vi "VI Linearisierung v2.vi"() -> ()   [LabVIEW 2020, in "Linearisierung v2.lvlib"] (continued)
      n15 = control-ref of="PrüfgasName 2"() -> (w61:refnum<vi>)
      n16 = control-ref of="PrüfgasName 3"() -> (w62:refnum<vi>)
      n17 = control-ref of="PrüfgasName 4"() -> (w63:refnum<vi>)
      n18 = control-ref of="PrüfgasName 5"() -> (w64:refnum<vi>)
      n19 = control-ref of="PrüfgasName 6"() -> (w65:refnum<vi>)
      n20 = control-ref of="PrüfgasName 7"() -> (w66:refnum<vi>)
      n21 = control-ref of="PrüfgasName 8"() -> (w67:refnum<vi>)
      n22 = control-ref of="PrüfgasName 9"() -> (w68:refnum<vi>)
      n23 = control-ref of="PrüfgasName 10"() -> (w69:refnum<vi>)
      n24 = Build Array ("Array erstellen")(w60, w61, w62, w63, w64, w65, w66, w67, w68, w69) -> (w50:refnum<vi>[])
      n25 = Build Array ("Array erstellen")(w74, w59, w58, w57, w56, w55, w54, w53, w52, w51) -> (w73:refnum<vi>[])
      n26 = control-ref of="Parameterkontrolle:"() -> (w97:refnum<vi>)
      n27 = control-ref of="Parameterkontrolle: 2"() -> (w98:refnum<vi>)
      n28 = control-ref of="Parameterkontrolle: 3"() -> (w99:refnum<vi>)
      n29 = control-ref of="Parameterkontrolle: 4"() -> (w100:refnum<vi>)
      n30 = control-ref of="Parameterkontrolle: 5"() -> (w101:refnum<vi>)
      n31 = control-ref of="Parameterkontrolle: 6"() -> (w102:refnum<vi>)
      n32 = control-ref of="Parameterkontrolle: 7"() -> (w103:refnum<vi>)
      n33 = control-ref of="Parameterkontrolle: 8"() -> (w104:refnum<vi>)
      n34 = control-ref of="Parameterkontrolle: 9"() -> (w105:refnum<vi>)
      n35 = control-ref of="Parameterkontrolle: 10"() -> (w106:refnum<vi>)
      n36 = control-ref of="Abfragen"() -> (w95:refnum<vi>)
      n37 = control-ref of="Abfragen 2"() -> (w94:refnum<vi>)
      n38 = control-ref of="Abfragen 3"() -> (w93:refnum<vi>)
      n39 = control-ref of="Abfragen 4"() -> (w92:refnum<vi>)
      n40 = control-ref of="Abfragen 5"() -> (w91:refnum<vi>)
      n41 = control-ref of="Abfragen 6"() -> (w90:refnum<vi>)
      n42 = control-ref of="Abfragen 7"() -> (w89:refnum<vi>)
      n43 = control-ref of="Abfragen 8"() -> (w88:refnum<vi>)
      n44 = control-ref of="Abfragen 9"() -> (w87:refnum<vi>)
      n45 = control-ref of="Abfragen 10"() -> (w86:refnum<vi>)
      n46 = control-ref of="auto Scan Points"() -> (w84:refnum<vi>)
      n47 = control-ref of="auto Scan Points 2"() -> (w83:refnum<vi>)
      n48 = control-ref of="auto Scan Points 3"() -> (w82:refnum<vi>)
      n49 = control-ref of="auto Scan Points 4"() -> (w81:refnum<vi>)
      n50 = control-ref of="auto Scan Points 5"() -> (w80:refnum<vi>)
      n51 = control-ref of="auto Scan Points 6"() -> (w79:refnum<vi>)
      n52 = control-ref of="auto Scan Points 7"() -> (w78:refnum<vi>)
      n53 = control-ref of="auto Scan Points 8"() -> (w77:refnum<vi>)
      n54 = control-ref of="auto Scan Points 9"() -> (w76:refnum<vi>)
      n55 = control-ref of="auto Scan Points 10"() -> (w75:refnum<vi>)
      n56 = control-ref of="Stufen Tabelle"() -> (w108:refnum<vi>)
      n57 = control-ref of="Stufen Tabelle 2"() -> (w109:refnum<vi>)
      n58 = control-ref of="Stufen Tabelle 3"() -> (w110:refnum<vi>)
      n59 = control-ref of="Stufen Tabelle 4"() -> (w111:refnum<vi>)
      n60 = control-ref of="Stufen Tabelle 5"() -> (w112:refnum<vi>)
      n61 = control-ref of="Stufen Tabelle 6"() -> (w113:refnum<vi>)
      n62 = control-ref of="Stufen Tabelle 7"() -> (w114:refnum<vi>)
      n63 = control-ref of="Stufen Tabelle 8"() -> (w115:refnum<vi>)
      n64 = control-ref of="Stufen Tabelle 9"() -> (w116:refnum<vi>)
      n65 = control-ref of="Stufen Tabelle 10"() -> (w117:refnum<vi>)
      n66 = Build Array ("Array erstellen")(w84, w83, w82, w81, w80, w79, w78, w77, w76, w75) -> (w72:refnum<vi>[])
      n67 = Build Array ("Array erstellen")(w95, w94, w93, w92, w91, w90, w89, w88, w87, w86) -> (w85:refnum<vi>[])
      n68 = Build Array ("Array erstellen")(w108, w109, w110, w111, w112, w113, w114, w115, w116, w117) -> (w107:refnum<vi>[])
      n69 = Build Array ("Array erstellen")(w97, w98, w99, w100, w101, w102, w103, w104, w105, w106) -> (w96:refnum<vi>[])
      n70 = for {
        tunnel: w72 -> [w118] mode=indexing
        n71 = property class="Bool. (strikt)"(reference=w118, "Value"=TRUE ("Wert")) -> (error out=w119:errorcluster)  [unwired: 1 in, 1 out]
        n72 = call <vilib>:"Clear Errors.vi"("error in (no error)"=w119) -> ()  [unwired: 5 in, 2 out]
      }
      n73 = control-ref of="Autolin Hovacal"() -> (w49:refnum<vi>)
      n74 = control-ref of="Bearbeiter"() -> (w71:refnum<vi>)
      n75 = control-ref of="EPA Auswertung"() -> (w47:refnum<vi>)
      n76 = control-ref of="Daten"() -> (w48:refnum<vi>)
      n77 = control-ref of="LIN Filename override"() -> (w42:refnum<vi>)
      n78 = control-ref of="EPA Filename override"() -> (w41:refnum<vi>)
      n79 = control-ref of="File Name LIN"() -> (w46:refnum<vi>)
      n80 = control-ref of="EPA Filename"() -> (w45:refnum<vi>)
      n81 = control-ref of="Gasnummer Generieren"() -> (w43:refnum<vi>)
      n82 = Bundle("File Name LIN"=w46, "EPA Filename"=w45) -> (w44:T101)  [unwired: 1 in]
      n83 = Bundle("LIN Filename override"=w42, "EPA Filename override"=w41) -> (w40:T102)  [unwired: 1 in]
    }
    frame #1 {
      w185 = u16 0 items=["---", "NO (350,3000) LP 191C", "NO2 (150) LP 191C (1of2)", "NO2 (2000) LP 191C (2of2)", "N2O (300) LP 191C (1of2)", "NH3 (300) LP 191C (1of2)", "NH3 (900,3000) LP 191C (2of2)", "HNCO (400) 191C", "H2O% (30) LP 191C", "Formaldehyde (70,500) LP 191C", "CO2 low% (4) LP 191C (2of2)", "CO2% (20) LP 191C (1of2)", "CO (700) LP 191C (1of3)", "CO% (1) LP 191C (2of3)", "Propylene (1000) LP 191C", "Aromatic HC C7 (500) LP 191C", "Ethylene (1000) LP 191C", "CH4 (250) LP 191C (1of2)", "CH4 (5000) LP 191C (2of2)", "Ethane (1000) LP 191C", "Acetylene (1000) LP 191C", "HNO2 (20) 191C", "MeOH (1000) 191C", "CO% (10) LP 191C (3of3)", "Formic Acid (100) 191C", "SO2 (500) LP 191C", "Acetaldehyde (1000) LP 191C", "COS (100) LP 191C", "1,3 butadiene (100) LP 191C", "Oil as Octane (200) LP 191C", "N2O (1000) LP 191C (2of2)", "Propane (200) LP 191C", "NO2 autorange (2000)", "CO autorange (100000)", "CH4 autorange (5000)", "NH3 autorange (3000)", "NOx autorange (3000)", "HCD (10000)", "NMHCD (10000)", "CO2% autorange (20)", "H2Oppm (300000)", "N2O autorange (1000)", "NMNEHCD (3000)", "Temp. Gascell", "Pressure Gascell", "sBeam@2500", "Temp. HL zu FT-IR", "Temp. HL Extern SP1", "Austrittstemp. FT-IR", "Temp. Schaltschrank", "Konstant 0", "Konstant 50", "Konstant 100", "AK DUMMY"] ("passive Komponente:")
      # "#RickQuickTest_Features"
      # "#STB_keep"
      # "#LIN_only_saved_Polynoms"
      # "#PDF_manu_MG"
      # "Daten aufzeichnen"
      # "LIN"
      # "init Analysatoren"
      # "immer auf dieser Seite bleiben ?!"
      # "#Option10xSpanAuto"
      n84 = control-ref of="Hauptregisterkarte"() -> (w211:refnum<vi>)
      n85 = control-ref of="SpanRegister"() -> (w271:refnum<vi>)
      n86 = call "FGV Spans abarbeiten.vi"("Aktion"=Aktion_FGV_Spans_abarbeiten."init") -> ("error out"=w153:errorcluster)  [unwired: 5 in, 5 out]
      n87 = control-ref of="Polynom"() -> (w142:refnum<vi>)
      n88 = control-ref of="Istwerte Abholen"() -> (w251:refnum<vi>)
      n89 = control-ref of="Istwerte löschen"() -> (w252:refnum<vi>)
      n90 = control-ref of="Alles löschen"() -> (w253:refnum<vi>)
      n91 = control-ref of="STARTEN"() -> (w254:refnum<vi>)
      n92 = control-ref of="Speichern LIN"() -> (w165:refnum<vi>)
      n93 = control-ref of="EPA PDF erzeugen"() -> (w164:refnum<vi>)
      n94 = control-ref of="LIN Filename override"() -> (w122:refnum<vi>)
      n95 = control-ref of="EPA Filename override"() -> (w121:refnum<vi>)
      n96 = control-ref of="Spanfactor"() -> (w151:refnum<vi>)
      n97 = control-ref of="Offset"() -> (w150:refnum<vi>)
      n98 = control-ref of="Span 1"() -> (w265:refnum<vi>)
      n99 = control-ref of="Span 2"() -> (w264:refnum<vi>)
      n100 = control-ref of="Span 3"() -> (w263:refnum<vi>)
      n101 = control-ref of="Span 4"() -> (w262:refnum<vi>)
      n102 = control-ref of="Span 5"() -> (w261:refnum<vi>)
      n103 = control-ref of="Span 6"() -> (w260:refnum<vi>)
      n104 = control-ref of="Span 7"() -> (w259:refnum<vi>)
      n105 = control-ref of="Span 8"() -> (w258:refnum<vi>)
      n106 = control-ref of="Span 9"() -> (w257:refnum<vi>)
      n107 = control-ref of="Span 10"() -> (w256:refnum<vi>)
      n108 = control-ref of="HovaCAL MFC1 Komponente:"() -> (w175:refnum<vi>)
      n109 = control-ref of="HovaCAL MFC2 Komponente:"() -> (w174:refnum<vi>)
      n110 = control-ref of="HovaCAL MFC3 Komponente:"() -> (w173:refnum<vi>)
      n111 = control-ref of="HovaCAL MFC4 Komponente:"() -> (w172:refnum<vi>)
      n112 = control-ref of="HovaCAL MFC5 Komponente:"() -> (w171:refnum<vi>)
      n113 = control-ref of="HovaCAL Pump1 Komponente:"() -> (w170:refnum<vi>)
      n114 = control-ref of="HovaCAL Pump2 Komponente:"() -> (w169:refnum<vi>)
      n115 = Build Array(w265, w264, w263, w262, w261, w260, w259, w258, w257, w256) -> (w296:refnum<vi>[])
      n116 = control-ref of="Gasnummer Generieren"() -> (w250:refnum<vi>)
      n117 = control-ref of="Gasnummer HovaCal Interface"() -> (w248:refnum<vi>)
      n118 = control-ref of="Gasnummer HovaCal"() -> (w249:refnum<vi>)
      n119 = control-ref of="Gasnummer LIN"() -> (w163:refnum<vi>)
      n120 = control-ref of="Gasnummer EPA"() -> (w162:refnum<vi>)
      n121 = Bundle("Spanfactor"=w151, "Offset"=w150, "Polynom"=w142) -> (w146:T103)  [unwired: 1 in]
      n122 = control-ref of="passive Komponente:"() -> (w186:refnum<vi>)
      n123 = Bundle("Hauptregisterkarte"=w211, "SpanRegister"=w271) -> (w212:T104)  [unwired: 1 in]
      n124 = Build Array(w251, w252, w253, w254, w165, w164, w122, w121) -> (w244:refnum<vi>[])
      n125 = call "ClusterReferernzenAufschluesseln.vi"("Cluster in"=w296) -> ("error out"=w287:errorcluster, "Analysatoren"=w166:refnum<vi>[], "Ring Gasflasche aktiv out"=w167:refnum<vi>[], "Ring Components out"=w288:refnum<vi>[])  [unwired: 7 in]
      n126 = call "FGV SpanEinstellungen.vi"("Aktion"=Aktion_FGV_SpanEinstellungen."RegisterRef", "error in (no error)"=w153, "RegisterRefs"=w212) -> ("error out"=w239:errorcluster)  [unwired: 4 in, 4 out]
      n127 = disable-structure shown="Aktiviert" {
        disable-tunnel: w165 -> [w303 _]
        disable-tunnel: w164 -> [w302 _]
        disable-tunnel: w163 -> [w301 w306]
        disable-tunnel: w162 -> [w300 w305]
        disable-tunnel: [w299 w304] -> w161
        disable-tunnel: w122 -> [w298 _]
        disable-tunnel: w121 -> [w297 _]
        frame Enabled {
          # "#LinV2_auto_singleSave"
          n128 = Build Array(w298, w297, w303, w302, w301, w300) -> (w299:refnum<vi>[])
        }
        frame Disabled {
          n129 = Build Array(w306, w305) -> (w304:refnum<vi>[])
        }
      }
      n130 = Build Array(w175, w174, w173, w172, w171, w170, w169) -> (w168:refnum<vi>[])
      n131 = Build Array (concatenate)(w168, w186, w288) -> (w187:refnum<vi>[])
      n132 = local write "passive Komponente:"(w185) -> ()
      n133 = Build Array(w250, w248, w249, w163, w162) -> (w243:refnum<vi>[])
      n134 = call "FGV Gasbottledefinition.vi"("Aktion"=Aktion_FGV_Gasbottledefinition."lesen") -> ("Gasflaschen Liste gesamt"=w286:T105[])  [unwired: 8 in, 2 out]
      n135 = call "FGV SpanEinstellungen.vi"("Aktion"=Aktion_FGV_SpanEinstellungen."laden", "error in (no error)"=w239) -> ("error out"=w266:errorcluster, "Punkte umkehren und PDF Optionen Cluster"=w201:T109)  [unwired: 5 in, 3 out]
      n136 = for {
        tunnel: w286 -> [w327]
        tunnel: w167 -> [w325] mode=indexing
        tunnel: [w325] -> w284 mode=indexing
        n137 = call "Gasflaschen Auswahl.vi"("Gasflaschen Liste gesamt"=w327, "Ring (Eingang)"=w325) -> ("error out"=w326:errorcluster)  [unwired: 7 in, 2 out]
        n138 = call <vilib>:"Clear Errors.vi"("error in (no error)"=w326) -> ()  [unwired: 5 in, 2 out]
      }
      n139 = Unbundle By Name(w201) -> ("Punkte umkehren"=w200:bool[], "PDF Optionen"=w199:T108)
      n140 = call "FGV Gasliste.vi"("Aktionen"=FGV_FT-IR_Gasliste_Aktionen."lesen") -> ("Aktuelle Gasliste gesamt"=w292:T48[])  [unwired: 8 in, 2 out]
      n141 = control-ref of="EPA Optionsfeld"() -> (w144:refnum<vi>)
      n142 = call "FGV Komponentenreferenzen verwalten.vi"("Referenzen"=w187, "error in (no error)"=w287, "Aktion"=Aktion_FGV_Komponentenreferenz_verwalten."Referenzen init") -> ("error out"=w289:errorcluster)  [unwired: 12 in]
      n143 = control-ref of="Polynomkoeffizienten"() -> (w141:refnum<vi>)
      n144 = control-ref of="Komponente Daten Gen"() -> (w245:refnum<vi>)
      n145 = control-ref of="Komponentenanzeige LIN"() -> (w246:refnum<vi>)
      n146 = control-ref of="Komponentenanzeige EPA"() -> (w247:refnum<vi>)
      n147 = control-ref of="Einheit"() -> (w192:refnum<vi>)
      n148 = control-ref of="Einheit Deviation"() -> (w191:refnum<vi>)
      n149 = control-ref of="Polynom-Ordnung"() -> (w149:refnum<vi>)
      n150 = control-ref of="Spanfactor LIN"() -> (w148:refnum<vi>)
      n151 = control-ref of="Offset LIN"() -> (w147:refnum<vi>)
      n152 = call "FGV SpanEinstellungen.vi"("Aktion"=Aktion_FGV_SpanEinstellungen."init", "error in (no error)"=w266) -> ("error out"=w268:errorcluster, "SpanInletClusterArray out"=w269:T19[])  [unwired: 5 in, 3 out]
      n153 = Build Array (concatenate)("---" ("String"), w292) -> (w294:T48[])
      n154 = control-ref of="EPA Optionsfeld"() -> (w160:refnum<vi>)
      n155 = control-ref of="Autolin Hovacal"() -> (w206:refnum<vi>)
      n156 = Build Array(w245, w246, w247) -> (w190:refnum<vi>[])
      n157 = Build Array(w192, w191) -> (w189:refnum<vi>[])
      n158 = call "FGV SpanEinstellungen.vi"("Aktion"=Aktion_FGV_SpanEinstellungen."schreiben", "error in (no error)"=w268, "SpanInletClusterArray in"=w269) -> ("error out"=w222:errorcluster, "SpanInletClusterArray out"=w223:T19[])  [unwired: 4 in, 3 out]
      n159 = control-ref of="Bearbeiter"() -> (w210:refnum<vi>)
      n160 = Bundle("Polynom-Ordnung"=w149, "Spanfactor LIN"=w148, "Offset LIN"=w147, "Polynomkoeffizienten"=w141) -> (w145:T110)  [unwired: 1 in]
      n161 = control-ref of="Modus"() -> (w204:refnum<vi>)
      n162 = call "FGV Komponentenreferenzen verwalten.vi"("Strings []"=w294, "error in (no error)"=w289, "Aktion"=Aktion_FGV_Komponentenreferenz_verwalten."Ring beschreiben") -> ("error out"=w214:errorcluster)  [unwired: 12 in]
      n163 = control-ref of="Kalibrierauswahl"() -> (w209:refnum<vi>)
      n164 = control-ref of="Conditions:"() -> (w208:refnum<vi>)
      n165 = control-ref of="HovaCAL AutoLin MFC"() -> (w207:refnum<vi>)
      n166 = Unbundle By Name(w199) -> ("PDF Einzelseiten Komponenten"=w152:bool, "PDF Einzelseiten Span"=w125:bool, "PDF Deckblatt"=w198:bool, "PDF öffnen"=w197:bool, "Graphik für Messwerte"=w129:bool)
      n167 = for {
        tunnel: w203 -> [w317] mode=indexing
        tunnel: w200 -> [w316] mode=indexing
        tunnel: [w315] -> w202 mode=indexing
        n168 = property class="Bool. (strikt)"(reference=w317, "Value"=w316) -> (reference out=w315:refnum<vi>, error out=w318:errorcluster)  [unwired: 1 in]
        n169 = call <vilib>:"Clear Errors.vi"("error in (no error)"=w318) -> ()  [unwired: 5 in, 2 out]
      }
      n170 = call "get first active SPAN.vi"("error in (no error)"=w222, "SpanInletClusterArray in"=w223) -> ("error out"=w220:errorcluster, "Index first active SPAN"=w219:i32, "SpanInletClusterArray out"=w221:T19[])  [unwired: 7 in]
      n171 = Build Array(w210, w160, w209, w208, w207, w206, w204) -> (w205:refnum<vi>[])
      n172 = Bundle(w190, w189, w146, w145, "EPA Optionsfeld"=w144) -> (w143:T111)  [unwired: 1 in]
      n173 = call "get SPAN first active component.vi"("error in (no error)"=w220, "SPAN Idx"=w219, "SpanInletClusterArray in"=w221) -> ("error out"=w213:errorcluster, "first aktive Komponente"=w216:i32, "SPAN Idx out"=w217:i32, "SpanInletClusterArray out"=w218:T19[])  [unwired: 5 in]
      n174 = control-ref of="post processing done"() -> (w178:refnum<vi>)
      n175 = control-ref of="post processing PDFs"() -> (w134:refnum<vi>)
      n176 = control-ref of="passive Komponente:"() -> (w188:refnum<vi>)
      n177 = control-ref of="post processing"() -> (w183:refnum<vi>)
      n178 = Build Array (concatenate)(w161, w160) -> (w159:refnum<vi>[])
      n179 = control-ref of="Eingabetabelle"() -> (w155:refnum<vi>)
      n180 = control-ref of="post processing done"() -> (w176:refnum<vi>)
      n181 = control-ref of="post processing PDFs"() -> (w133:refnum<vi>)
      n182 = call "Set actual ProtocolData from SPAN.vi"("Punkte umkehren Array"=w202, "error in (no error)"=w213, "Comp Idx"=w216, "Index in"=w217, "SpanInletClusterArray in"=w218) -> ("error out"=w156:errorcluster, "SpanInletClusterArray out"=w158:T19[])  [unwired: 3 in, 2 out]
      n183 = control-ref of="post processing"() -> (w179:refnum<vi>)
      n184 = Bundle("passive Komponente:"=w188, "post processing"=w183, "post processing done"=w178, "post processing PDFs"=w134) -> (w184:T112)  [unwired: 1 in]
      n185 = call "FGV SPAN Verriegelung.vi"("Processing Cluster"=w184, "Lin Param Elements Array"=w205, "aktion"=Aktion_FGV_SPAN_Verriegelung."setrefs", "error in (no error)"=w239, "Components Array"=w243, "Buttons Array"=w244, "Set Component Cluster"=w143) -> ("error out"=w240:errorcluster)  [unwired: 2 in, 2 out]
      n186 = call "Init Tables.vi"("error in (no error)"=w156, "Eingabetabelle"=w155, "Index in"=0, "SpanInletClusterArray in"=w158) -> ("SpanInletCluster out"=w157:T19[])  [unwired: 4 in, 3 out]
      n187 = call "FGV SPAN Verriegelung.vi"("aktion"=Aktion_FGV_SPAN_Verriegelung."unlock", "error in (no error)"=w240) -> ("error out"=w139:errorcluster)  [unwired: 7 in, 2 out]
      n188 = Select(t=w129, s=w125, f=T1 FALSE ("t")) -> (s? t:f=w130:T1)
      n189 = for {
        tunnel: w284 -> [w323] mode=indexing
        tunnel: w157 -> [w322] mode=indexing
        shift-right: [w320] -> w215
        shift-left: w214 -> [w319]
        n190 = Unbundle By Name(w322) -> ("Konfig Gasflasche"=w321:T20)
        n191 = call "Konfig Gasflasche aktiv.vi"("error in (no error)"=w319, "Konfig Gasflasche"=w321, "Referenz Gasflasche"=w323) -> ("error out"=w324:errorcluster)  [unwired: 8 in]
        n192 = call <vilib>:"Clear Errors.vi"("error in (no error)"=w324) -> ("error out"=w320:errorcluster)  [unwired: 5 in, 1 out]
      }
      n193 = call "FGV Gasteilerliste laden.vi"("Aktion"=Aktion_FGV_Gasteilerliste_laden."laden", "error in (no error)"=w215) -> ("error out"=w224:errorcluster)  [unwired: 7 in, 2 out]
      n194 = call "FGV Gasteilerliste laden.vi"("Aktion"=Aktion_FGV_Gasteilerliste_laden."Liste erstellen", "error in (no error)"=w224) -> ("error out"=w237:errorcluster)  [unwired: 7 in, 2 out]
      n195 = call "get Summenformeln and update.vi"("Fehler (Eingang, kein Fehler)"=w237, "SpanInletClusterArray in"=w223) -> ("error out"=w193:errorcluster, "ident"=w196:bool, "Summenformeln 1.Komponente"=w236:T12[], "SpanInletClusterArray out"=w195:T19[])  [unwired: 6 in]
      n196 = case shown="False" w196 {
        tunnel: w195 -> [w311 w314]
        tunnel: [w309 w314] -> w194
        tunnel: w193 -> [w307 _]
        frame False {
          n197 = call "FGV SpanEinstellungen.vi"("Aktion"=Aktion_FGV_SpanEinstellungen."schreiben", "error in (no error)"=w307, "SpanInletClusterArray in"=w311) -> ("error out"=w308:errorcluster, "SpanInletClusterArray out"=w310:T19[])  [unwired: 4 in, 3 out]
          n198 = call "FGV SpanEinstellungen.vi"("Aktion"=Aktion_FGV_SpanEinstellungen."speichern", "error in (no error)"=w308, "SpanInletClusterArray in"=w310) -> ("SpanInletClusterArray out"=w309:T19[])  [unwired: 4 in, 4 out]
        }
        frame True {
        }
      }
      n199 = Bundle("post processing"=w179, "post processing done"=w176, "post processing PDFs"=w133) -> (w177:T113)  [unwired: 1 in]
      n200 = call "FGV Post Processing.vi"("LIN/EPA Refs Array"=w159, "Aktion"=Aktion_FGV_Post_Processing."set ref", "Refs Cluster"=w177) -> ("error out"=w180:errorcluster)  [unwired: 5 in, 3 out]
      n201 = local write "PDF single pages Components"(w152) -> ()
      n202 = local write "PDF single pages Span"(w125) -> ()
      n203 = local write "PDF Deckblatt"(w198) -> ()
      n204 = local write "PDF öffnen"(w197) -> ()
      n205 = local write "Graphik für Messwerte"(w130) -> ()
      n206 = call "LIN Polynom Ordnung je Komponente für Protokoll.vi"("Aktion"=Aktion_LIN_Polynom_Ordnung_je_Komponente_für_Protokoll."init initial", "error in (no error)"=w139, "Index in"=T69 {"active SPAN Idx"=0, "active Component Index"=0}) -> ("error out"=w136:errorcluster)  [unwired: 2 in, 6 out]
      n207 = call "FGV Post Processing.vi"("Aktion"=Aktion_FGV_Post_Processing."reset", "error in (no error)"=w180) -> ()  [unwired: 6 in, 4 out]
      n208 = call "LIN Polynom Ordnung oder Aktiv Changes für Postprocessing.vi"("Aktion"=Aktion_LIN_Polynom_Ordnung_ode_Aktiv_Changes_für_Postprocessing."init initial", "error in (no error)"=w136, "active SPAN Idx"=0) -> ("error out"=w132:errorcluster)  [unwired: 5 in, 3 out]
      n209 = call "FGV SPAN Stufentabellen.vi"("Aktion"=Aktion_FGV_SPAN_Stufentabellen."init", "error in (no error)"=w132) -> ()  [unwired: 5 in, 4 out]
      n210 = Index Array(array=w194) -> (element #1=w281:T19, element #2=w280:T19, element #3=w279:T19, element #4=w278:T19, element #5=w277:T19, element #6=w276:T19, element #7=w275:T19, element #8=w274:T19, element #9=w273:T19, element #10=w272:T19)  [unwired: 10 in]
      n211 = Index Array(array=w236) -> (element #1=w235:T12, element #2=w234:T12, element #3=w233:T12, element #4=w232:T12, element #5=w231:T12, element #6=w230:T12, element #7=w229:T12, element #8=w228:T12, element #9=w227:T12, element #10=w226:T12)  [unwired: 10 in]
      n212 = Select(t=T66."Enabled", s=w125, f=T66."Disabled and Grayed Out" ("Deaktiviert")) -> (s? t:f=w123:T66)
      n213 = property on="Graphik für Messwerte" class="Bool. (strikt)"("DisabledEnum"=w123) -> (error out=w124:errorcluster)  [unwired: 2 in, 1 out]
      n214 = local write "Span 1"(w281) -> ()
      n215 = local write "Span 2"(w280) -> ()
      n216 = local write "Span 3"(w279) -> ()
      n217 = local write "Span 4"(w278) -> ()
      n218 = local write "Span 5"(w277) -> ()
      n219 = local write "Span 6"(w276) -> ()
      n220 = local write "Span 7"(w275) -> ()
      n221 = local write "Span 8"(w274) -> ()
      n222 = local write "Span 9"(w273) -> ()
      n223 = local write "Span 10"(w272) -> ()
      n224 = local write "PrüfgasName"(w235) -> ()
      n225 = local write "PrüfgasName 2"(w234) -> ()
      n226 = local write "PrüfgasName 3"(w233) -> ()
      n227 = local write "PrüfgasName 4"(w232) -> ()
      n228 = local write "PrüfgasName 5"(w231) -> ()
      n229 = local write "PrüfgasName 6"(w230) -> ()
      n230 = local write "PrüfgasName 7"(w229) -> ()
      n231 = local write "PrüfgasName 8"(w228) -> ()
      n232 = local write "PrüfgasName 9"(w227) -> ()
      n233 = local write "PrüfgasName 10"(w226) -> ()
      n234 = call <vilib>:"Clear Errors.vi"("error in (no error)"=w124) -> ()  [unwired: 5 in, 2 out]
    }
    frame #2 {
      w373 = FALSE  # sofort HovaCALInterface-Freigabe
      # "#SystemEinstellungenV2 #HovaCALInterface #HovaCALMultiMFC"
      n235 = control-ref of="MFC Output 0"() -> (w336:refnum<vi>)
      n236 = control-ref of="MFC Output 1"() -> (w335:refnum<vi>)
      n237 = control-ref of="MFC Output 2"() -> (w334:refnum<vi>)
      n238 = control-ref of="MFC Output 3"() -> (w333:refnum<vi>)
      n239 = control-ref of="MFC Output 4"() -> (w332:refnum<vi>)
      n240 = control-ref of="Pump Output 1"() -> (w355:refnum<vi>)
      n241 = control-ref of="Pump Output 2"() -> (w354:refnum<vi>)
      n242 = control-ref of="MFC0"() -> (w363:refnum<vi>)
      n243 = control-ref of="MFC1"() -> (w362:refnum<vi>)
      n244 = control-ref of="MFC2"() -> (w361:refnum<vi>)
      n245 = control-ref of="MFC3"() -> (w349:refnum<vi>)
      n246 = control-ref of="MFC4"() -> (w348:refnum<vi>)
      n247 = control-ref of="Pump 1"() -> (w359:refnum<vi>)
      n248 = control-ref of="Pump 2"() -> (w358:refnum<vi>)
      n249 = Build Array(w359, w358) -> (w356:refnum<vi>[])
      n250 = Build Array(w363, w362, w361, w349, w348) -> (w360:refnum<vi>[])
      n251 = control-ref of="Konfig Gasteiler"() -> (w330:refnum<vi>)
      n252 = Build Array(w336, w335, w334, w333, w332) -> (w331:refnum<vi>[])
      n253 = Build Array(w355, w354) -> (w353:refnum<vi>[])
      n254 = call "FGV_HovaCAL_Interface_Kommandos.vi"("Aktion"=Aktion_FGV_HovaCAL_Interface_Kommandos."lesen") -> ("gesammelt ?"=w371:bool)  [unwired: 4 in, 5 out]
      n255 = property on="HovaCALInterface-Freigabe" class="Bool."("Visible"=w371) -> (error out=w370:errorcluster)  [unwired: 2 in, 1 out]
      n256 = call "Gasteiler initialisieren.vi"("Gasteiler Referenz"=w330) -> ()  [unwired: 11 in]
      n257 = call <vilib>:"Clear Errors.vi"("error in (no error)"=w370) -> ()  [unwired: 5 in, 2 out]
      n258 = control-ref of="HovaCAL MFC Gase Cluster 1"() -> (w369:refnum<vi>)
      n259 = control-ref of="HovaCAL MFC Gase Cluster 2"() -> (w368:refnum<vi>)
      n260 = control-ref of="HovaCAL MFC Gase Cluster 3"() -> (w367:refnum<vi>)
      n261 = control-ref of="HovaCAL MFC Gase Cluster 4"() -> (w366:refnum<vi>)
      n262 = control-ref of="HovaCAL MFC Gase Cluster 5"() -> (w365:refnum<vi>)
      n263 = control-ref of="fix+MFC1"() -> (w340:refnum<vi>)
      n264 = control-ref of="fix+MFC2"() -> (w341:refnum<vi>)
      n265 = control-ref of="fix+MFC3"() -> (w342:refnum<vi>)
      n266 = control-ref of="fix+MFC4"() -> (w343:refnum<vi>)
      n267 = control-ref of="fix+MFC5"() -> (w344:refnum<vi>)
      n268 = control-ref of="fix+Pump1"() -> (w345:refnum<vi>)
      n269 = control-ref of="fix+Pump2"() -> (w346:refnum<vi>)
      n270 = control-ref of="Hauptregisterkarte"() -> (w351:refnum<vi>)
      n271 = control-ref of="Cluster.PumpModeGeneral-Cluster"() -> (w381:refnum<vi>)
      n272 = control-ref of="Cluster.Flow Output Cluster (Ausgang)"() -> (w380:refnum<vi>)
      n273 = control-ref of="Cluster.PumpModeGeneral-Cluster 2"() -> (w328:refnum<vi>)
      n274 = control-ref of="HovaCAL Limits Cluster"() -> (w388:refnum<vi>)
      n275 = control-ref of="HovaCAL SetPumpMode"() -> (w387:refnum<vi>)
      n276 = control-ref of="HovaCAL Cluster.PumpModeGeneral"() -> (w386:refnum<vi>)
      n277 = control-ref of="HovaCAL Flow Input Cluster"() -> (w385:refnum<vi>)
      n278 = control-ref of="System Cluster"() -> (w377:refnum<vi>)
      n279 = control-ref of="Cluster.Temp Cluster"() -> (w382:refnum<vi>)
      n280 = control-ref of="Cluster.Pump MassFlow-Cluster"() -> (w379:refnum<vi>)
      n281 = control-ref of="HovaCAL SetPumpMode-Cluster"() -> (w374:refnum<vi>)
      n282 = control-ref of="HovaCAL Temperature"() -> (w384:refnum<vi>)
      n283 = control-ref of="MFC Flow Cluster"() -> (w376:refnum<vi>)
      n284 = control-ref of="HovaCAL AutoLin MFC"() -> (w383:refnum<vi>)
      n285 = Build Array(w369, w368, w367, w366, w365) -> (w364:refnum<vi>[])
      n286 = Build Array(w340, w341, w342, w343, w344, w345, w346) -> (w338:refnum<vi>[])
      n287 = Bundle("System Cluster"=w377, "MFC Flow Cluster"=w376) -> (w375:T114)  [unwired: 1 in]
      n288 = Bundle ("Bündeln")(w331, "Cluster.Temp Cluster"=w382, "Cluster.PumpModeGeneral-Cluster"=w381, w353, "Cluster.Flow Output Cluster (Ausgang)"=w380, "Cluster.Pump MassFlow-Cluster"=w379, "Cluster.PumpModeGeneral-Cluster 2"=w328) -> (w329:T115)  [unwired: 1 in]
      n289 = Bundle("HovaCAL Limits Cluster"=w388, "HovaCAL SetPumpMode"=w387, "HovaCAL Cluster.PumpModeGeneral"=w386, "HovaCAL SetPumpMode-Cluster"=w374, "HovaCAL Flow Input Cluster"=w385, w360, "HovaCAL Temperature"=w384, w356, "HovaCAL AutoLin MFC"=w383, w364) -> (w357:T116)  [unwired: 1 in]
      n290 = property class="RKElem (strikt)"(reference=w351) -> (error out=w352:errorcluster, "Pages"=w350:refnum<vi>[])  [unwired: 1 in, 1 out]
      n291 = Bundle(w339, w338) -> (w337:cluster{refnum<vi>[], refnum<vi>[]})  [unwired: 1 in]
      n292 = call "FGV_HovaCAL_Interface_ControlReferenzen.vi"("Aktion"=enum16{"lesen", "schreiben"}."schreiben", "MFC fix Cluster"=w337, "System Cluster"=w375, "Set Cluster"=w357, "Get Cluster"=w329) -> ("Fehler (Ausgang)"=w347:errorcluster)  [unwired: 2 in, 4 out]
      n293 = for {
        tunnel: w352 -> [w400]
        tunnel: w350 -> [w397] mode=indexing
        n294 = property class="Seite"(reference=w397, error in=w400, "PageVis"=TRUE ("Seite sichtbar")) -> (error out=w398:errorcluster)  [unwired: 1 out]
        n295 = call <vilib>:"Clear Errors.vi"("error in (no error)"=w398) -> ()  [unwired: 5 in, 2 out]
      }
      n296 = disable-structure shown="TestRun==TRUE" {
        disable-tunnel: w347 -> [w391 _]
        frame condition #0 (active) {
          n297 = call "TestRun HovaCAL SystemValues.vi"() -> ("Info Cluster"=w389:T117)  [unwired: 11 in]
          n298 = stacked-sequence {
            tunnel: w389 -> [w393 w395]
            tunnel: [w392 _] -> w390
            frame #0 {
              n299 = call "FGV_HovaCAL_Interface_GetData.vi"("Aktion"=Aktion_FGV_HovaCAL_Interface_GetData."SystemInfo", "System Cluster in"=w393) -> ("System Cluster out"=w392:T117)  [unwired: 5 in, 4 out]
            }
            frame #1 {
              n300 = call "FGV_HovaCAL_Interface_SetData.vi"("System Cluster in"=w395, "Aktion"=Aktion_FGV_HovaCAL_Interface_SetData."init") -> ()  [unwired: 7 in, 7 out]
            }
          }
          n301 = call "Init_Controls.vi"("Fehler (Eingang, kein Fehler)"=w391, "Info Cluster"=w390) -> ()  [unwired: 8 in, 2 out]
        }
        frame condition #1 {
        }
      }
    }
    frame #3 {
      # "#HovaCALInterface"
      n302 = call "FGV Gasteiler.vi"("Aktionen"=Aktionen_FGV_Gasteiler_Daten."lesen") -> ("Gasteiler Daten"=w412:T118)  [unwired: 11 in, 7 out]
      n303 = Unbundle By Name(w412) -> ("Gasteiler"=w410:T12, "Gasteiler Stufen"=w409:T16, "Gasteiler Type"=w408:T15, "Gasteiler Span Eingänge"=w407:u16)
      n304 = disable-structure shown="EPA_aktiv==FALSE" {
        frame condition #0 (active) {
          n305 = control-ref of="Hauptregisterkarte"() -> (w507:refnum<vi>)
          n306 = property class="RKElem (strikt)"(reference=w507) -> (error out=w508:errorcluster, "Pages"=w506:refnum<vi>[])  [unwired: 1 in, 1 out]
          n307 = To Word Integer(number=T8."EPA 1065-307" ("Hauptregisterkarte")) -> (16bit integer=w509:i16)
          n308 = Index Array(array=w506, index=w509) -> (element=w505:refnum<vi>)
          n309 = property class="Seite"(reference=w505, error in=w508, "PageVis"=TRUE ("Seite sichtbar")) -> (error out=w503:errorcluster)  [unwired: 1 out]
          n310 = call <vilib>:"Clear Errors.vi"("error in (no error)"=w503) -> ()  [unwired: 5 in, 2 out]
        }
        frame condition #1 {
          n311 = control-ref of="Hauptregisterkarte"() -> (w515:refnum<vi>)
          n312 = property class="RKElem (strikt)"(reference=w515) -> (error out=w516:errorcluster, "Pages"=w514:refnum<vi>[])  [unwired: 1 in, 1 out]
          n313 = To Word Integer(number=T8."EPA 1065-307" ("Hauptregisterkarte")) -> (16bit integer=w517:i16)
          n314 = Index Array(array=w514, index=w517) -> (element=w513:refnum<vi>)
          n315 = property class="Seite"(reference=w513, error in=w516, "PageVis"=FALSE ("Seite sichtbar")) -> (error out=w511:errorcluster)  [unwired: 1 out]
          n316 = call <vilib>:"Clear Errors.vi"("error in (no error)"=w511) -> ()  [unwired: 5 in, 2 out]
        }
      }
      n317 = disable-structure shown="BullZip==TRUE" {
        frame condition #0 (active) {
          w500 = TRUE ("Sichtbar")
          n318 = property on="EPA Filename" class="Str (strikt)"("Visible"=w500) -> (error out=w499:errorcluster)  [unwired: 2 in, 1 out]
          n319 = property on="EPA Pfad" class="Pfad (strikt)"("Visible"=w500) -> (error out=w498:errorcluster)  [unwired: 2 in, 1 out]
          n320 = Merge Errors(w499, w498) -> (w497:errorcluster)
          n321 = call <vilib>:"Clear Errors.vi"("error in (no error)"=w497) -> ()  [unwired: 5 in, 2 out]
        }
        frame condition #1 {
          w501 = TRUE ("Sichtbar")
          n322 = property on="EPA Filename" class="Str (strikt)"("Visible"=w501) -> ()  [unwired: 2 in, 2 out]
          n323 = property on="EPA Pfad" class="Pfad (strikt)"("Visible"=w501) -> ()  [unwired: 2 in, 2 out]
        }
      }
      n324 = local write "Gasteiler"(w410) -> ()
      n325 = local write "Gasteiler Stufen"(w409) -> ()
      n326 = local write "Gasteiler Type"(w408) -> ()
      n327 = local write "Gasteiler Span Eingänge"(w407) -> ()
      n328 = call "Lin Daten aufarbeiten.vi"("Aktionen"=Aktion_Lin_Daten_aufarbeiten."lesen") -> ("Lin-Polynom"=w455:T119)  [unwired: 16 in, 10 out]
      n329 = call "FGV Gasteiler.vi"("Aktionen"=Aktionen_FGV_Gasteiler_Daten."lesen") -> ("Gasteiler Daten"=w447:T118)  [unwired: 11 in, 7 out]
      n330 = control-ref of="Hauptregisterkarte"() -> (w451:refnum<vi>)
      n331 = Unbundle By Name(w455) -> ("HovaCAL Flow AutoLin"=w417:T33, "Conditions:"=w423:T59, "EPA Optionsfeld"=w402:T2, "Bearbeiter/in"=w454:string, "Autolin Hovacal"=w420:T61, "Kalibrierauswahl"=w431:T5, "Lin Modus"=w406:T10)
      n332 = Unbundle By Name(w447) -> ("Gasteiler Type"=w446:T15)
      n333 = disable-structure shown="FID==TRUE" {
        frame condition #0 {
          w489 = TRUE
          n334 = property on="FID 0 kalibrieren" class="Bool."("Visible"=w489) -> (error out=w491:errorcluster)  [unwired: 2 in, 1 out]
          n335 = property on="FID E kalibrieren" class="Bool."("Visible"=w489) -> (error out=w490:errorcluster)  [unwired: 2 in, 1 out]
          n336 = Merge Errors(w491, w490) -> (w492:errorcluster)
          n337 = call <vilib>:"Clear Errors.vi"("error in (no error)"=w492) -> ()  [unwired: 5 in, 2 out]
        }
        frame condition #1 (active) {
          w493 = FALSE
          n338 = property on="FID 0 kalibrieren" class="Bool."("Visible"=w493) -> (error out=w495:errorcluster)  [unwired: 2 in, 1 out]
          n339 = property on="FID E kalibrieren" class="Bool."("Visible"=w493) -> (error out=w494:errorcluster)  [unwired: 2 in, 1 out]
          n340 = Merge Errors(w495, w494) -> (w496:errorcluster)
          n341 = call <vilib>:"Clear Errors.vi"("error in (no error)"=w496) -> ()  [unwired: 5 in, 2 out]
        }
      }
      n342 = To Unsigned Word Integer(number=LinV2_Registerkarten."Einstellungen" ("Hauptregisterkarte")) -> (unsigned 16bit integer=w441:u16)
      n343 = To Word Integer(number=T8."HovaCal Einstellungen" ("Hauptregisterkarte")) -> (16bit integer=w416:i16)
      n344 = To Word Integer(number=T8."HovaCAL Interface" ("Hauptregisterkarte")) -> (16bit integer=w415:i16)
      n345 = property class="RKElem (strikt)"(reference=w451) -> (error out=w422:errorcluster, "Pages"=w450:refnum<vi>[])  [unwired: 1 in, 1 out]
      n346 = local write "HovaCAL Flow AutoLin"(w417) -> ()
      n347 = Not Equal To 0?(x=w431) -> (x != 0?=w430:bool)
      n348 = local write "Hauptregisterkarte"(w441) -> ()
      n349 = local write "Modus"(w406) -> ()
      n350 = local write "Conditions:"(w423) -> ()
      n351 = local write "Bearbeiter"(w454) -> ()
      n352 = local write "Kalibrierauswahl"(w431) -> ()
      n353 = property on="Start LinCheck" class="Bool."("Visible"=w430) -> (error out=w432:errorcluster)  [unwired: 2 in, 1 out]
      n354 = disable-structure shown="Aktiviert" {
        disable-tunnel: w402 -> [_ w458]
        disable-tunnel: [EPA_Optionsfeld."Istwert" ("EPA Optionsfeld") w458] -> w401
        frame Enabled {
          # "#EPA_immer_Istwerte"
        }
        frame Disabled {
        }
      }
      n355 = Equal?(x=Gasteiler_Type."HovaCal", y=w446) -> (x = y?=w421:bool)
      n356 = disable-structure shown="HovaCALInterface==TRUE, Standard" {
        disable-tunnel: [w479 w480] -> w440
        disable-tunnel: w421 -> [w478 w480]
        frame condition #0 {
          n357 = Not(x=w478) -> (.not. x?=w479:bool)
        }
        frame condition #1 (active) {
        }
      }
      n358 = call "FGV Stoerungen sammeln und auswerten.vi"("Aktion"=Aktion_FGV_Stoerungen_sammeln_und_auswerten."init") -> ("error out"=w403:errorcluster)  [unwired: 12 in, 6 out]
      n359 = Index Array(array=w450, index #1=w416, index #2=w415) -> (element #1=w449:refnum<vi>, element #2=w419:refnum<vi>)
      n360 = disable-structure shown="HovaCALInterface==TRUE, Standard" {
        disable-tunnel: w420 -> [w475 w477]
        frame condition #0 (active) {
          n361 = call "FGV_HovaCAL_Interface_AutoLin_MFC.vi"("Aktion"=enum16{"lesen", "schreiben"}."schreiben", "AutoLin MFC"=w475) -> ("error out"=w473:errorcluster)  [unwired: 6 in, 3 out]
          n362 = call "FGV_HovaCAL_Interface_AutoLin_MFC.vi"("Aktion"=Aktion_FGV_HovaCAL_Interface_Autolin."init", "error in (no error)"=w473) -> ()  [unwired: 6 in, 4 out]
        }
        frame condition #1 {
          n363 = local write "Autolin Hovacal"(w477) -> ()
        }
      }
      n364 = disable-structure shown="HovaCALInterface==TRUE" {
        disable-tunnel: w449 -> [w465 w472]
        disable-tunnel: [w464 w471] -> w439
        disable-tunnel: w422 -> [w463 w470]
        disable-tunnel: w421 -> [w462 w466]
        disable-tunnel: w419 -> [w461 w469]
        disable-tunnel: [w459 w468] -> w418
        frame condition #0 {
          n365 = property class="Seite"(reference=w465, error in=w463, "PageVis"=w462) -> (error out=w464:errorcluster)  [unwired: 1 out]
          n366 = property class="Seite"(reference=w461, "PageVis"=FALSE ("Seite sichtbar")) -> (error out=w459:errorcluster)  [unwired: 1 in, 1 out]
        }
        frame condition #1 (active) {
          n367 = property class="Seite"(reference=w472, error in=w470, "PageVis"=FALSE ("Seite sichtbar")) -> (error out=w471:errorcluster)  [unwired: 1 out]
          n368 = property class="Seite"(reference=w469, "PageVis"=w466) -> (error out=w468:errorcluster)  [unwired: 1 in, 1 out]
        }
      }
      n369 = property on="parity" class="Ring (strikt)"("Visible"=w440) -> (error out=w438:errorcluster)  [unwired: 2 in, 1 out]
      n370 = property on="stop bits" class="Ring (strikt)"("Visible"=w440) -> (error out=w437:errorcluster)  [unwired: 2 in, 1 out]
      n371 = property on="Baud Rate" class="Ring (strikt)"("Visible"=w440) -> (error out=w436:errorcluster)  [unwired: 2 in, 1 out]
      n372 = property on="flow control" class="Ring (strikt)"("Visible"=w440) -> (error out=w435:errorcluster)  [unwired: 2 in, 1 out]
      n373 = property on="data bits" class="Ring (strikt)"("Visible"=w440) -> (error out=w434:errorcluster)  [unwired: 2 in, 1 out]
      n374 = local write "EPA Optionsfeld"(w401) -> ()
      n375 = call "FGV Rohmesswerte sammeln.vi"("error in (no error)"=w403, "Aktion"=Aktion_FGV_Rohmesswerte_sammeln."löschen") -> ()  [unwired: 10 in, 4 out]
      n376 = disable-structure shown="PMA==TRUE" {
        frame condition #0 {
          w481 = TRUE
          n377 = property on="PMD 0 kalibrieren" class="Bool."("Visible"=w481) -> (error out=w483:errorcluster)  [unwired: 2 in, 1 out]
          n378 = property on="PMD  E kalibrieren" class="Bool."("Visible"=w481) -> (error out=w482:errorcluster)  [unwired: 2 in, 1 out]
          n379 = Merge Errors(w483, w482) -> (w484:errorcluster)
          n380 = call <vilib>:"Clear Errors.vi"("error in (no error)"=w484) -> ()  [unwired: 5 in, 2 out]
        }
        frame condition #1 (active) {
          w485 = FALSE
          n381 = property on="PMD 0 kalibrieren" class="Bool."("Visible"=w485) -> (error out=w487:errorcluster)  [unwired: 2 in, 1 out]
          n382 = property on="PMD  E kalibrieren" class="Bool."("Visible"=w485) -> (error out=w486:errorcluster)  [unwired: 2 in, 1 out]
          n383 = Merge Errors(w487, w486) -> (w488:errorcluster)
          n384 = call <vilib>:"Clear Errors.vi"("error in (no error)"=w488) -> ()  [unwired: 5 in, 2 out]
        }
      }
      n385 = control-ref of="Eingabetabelle"() -> (w453:refnum<vi>)
      n386 = Merge Errors(w432, w439, w418, w438, w437, w436, w435, w434) -> (w433:errorcluster)
      n387 = call "Editierte Zelle merken.vi"("Aktion"=enum16{"init", "lesen", "schreiben"}."init", "Eingabetabelle"=w453) -> ()  [unwired: 8 in, 2 out]
      n388 = call <vilib>:"Clear Errors.vi"("error in (no error)"=w433) -> ()  [unwired: 5 in, 2 out]
      n389 = control-ref of="Gase"() -> (w443:refnum<vi>)
      n390 = property on="Aufschaltung CalGas" class="Cluster (strikt)"() -> (error out=w427:errorcluster, "Controls[]"=w428:refnum<vi>[])  [unwired: 2 in, 1 out]
      n391 = call "FGV CalGas.vi"("Aktionen"=FGV_CalGas_Aktionen."KAL extrahieren") -> ("Def.CalGas"=w429:T123)  [unwired: 6 in, 4 out]
      n392 = call "FGV_Betreibsdaten.vi"("Gase"=w443, "Enum"=Aktion_FGV_Betriebsdaten."GaseRef") -> ()  [unwired: 10 in, 8 out]
      n393 = call "FGV Span.vi"("Aktion"=Aktion_FGV_Span."Seite aktiv", "Aktiv"=TRUE) -> ()  [unwired: 6 in, 4 out]
      n394 = call "CalGas Auswahl - Strings zuweisen.vi"() -> ()  [unwired: 11 in, 1 out]
      n395 = call "CalGas Auswahl - Strings zuweisen.vi"("Def.CalGas"=w429, "Aufschaltung CalGas"=w428) -> ()  [unwired: 9 in, 1 out]
      n396 = call <vilib>:"Clear Errors.vi"("error in (no error)"=w427) -> ()  [unwired: 5 in, 2 out]
    }
    frame #4 {
      w518 = T9 path "D:/IAG_DATA/Log" ("Pfad Auto Lin")
      w531 = TRUE  # init
      w539 = T15 4 items=["LCD-Touch-Display", "Analog-Display", "AVL GDU", "Horiba GDC", "HovaCal", "Horiba 710 c"] ("x")
      w540 = T15 0 items=["LCD-Touch-Display", "Analog-Display", "AVL GDU", "Horiba GDC", "HovaCal", "Horiba 710 c"] ("x")
      w579 = T15 5 items=["LCD-Touch-Display", "Analog-Display", "AVL GDU", "Horiba GDC", "HovaCal", "Horiba 710 c"] ("x")
      w570 = T48 "" ("Status")
      w568 = u8 1
      w611 = u8 0
      w621 = T66."Enabled" ("Deaktiviert")
      # "#LinEinheiten"
      n397 = call "FGV Gasteiler.vi"("Aktionen"=Aktionen_FGV_Gasteiler_Daten."lesen") -> ("Gasteiler Daten"=w622:T118, "TCP"=w618:T128, "Serielle Parameter"=w585:T129, "error out"=w544:errorcluster)  [unwired: 11 in, 4 out]
      n398 = disable-structure shown="LINMultiSpan==TRUE" {
        disable-tunnel: [FALSE TRUE] -> w519
        frame condition #0 {
          # "#Linearisierung_PDF_Einstellungen_fix"
          n399 = call "FGV Post Processing.vi"("Aktion"=Aktion_FGV_Post_Processing."disable") -> ()  [unwired: 7 in, 4 out]
        }
        frame condition #1 (active) {
          n400 = call "FGV Post Processing.vi"("Aktion"=Aktion_FGV_Post_Processing."disable") -> ()  [unwired: 7 in, 4 out]
        }
      }
      n401 = disable-structure shown="HovaCALInterface==TRUE, Standard" {
        disable-tunnel: w585 -> [w628 _]
        frame condition #0 {
          # "#NeueLin_Bug Hovacal"
          n402 = Unbundle By Name(w628) -> ("VISA resource name"=w627:refnum<visa-resource-name>)
          n403 = call "FGV_Kommunikation.vi"("Aktion"=Aktion_FGV_Kom."Com ändern", "VISA"=w627) -> ("error out"=w630:errorcluster)  [unwired: 5 in, 4 out]
          n404 = call <vilib>:"Clear Errors.vi"("error in (no error)"=w630) -> ()  [unwired: 5 in, 2 out]
        }
        frame condition #1 (active) {
          # "#HovaCALInterface"
          n405 = call "FGV_HovaCAL_Interface_Kommandos.vi"("Aktion"=Aktion_FGV_HovaCAL_Interface_Kommandos."on top", "Kommando in"=Aktion_FGV_HovaCAL_Interface_Kommunikation."Com ändern" ("Kommando")) -> ()  [unwired: 3 in, 6 out]
        }
      }
      n406 = call "Polynom Daten speichern.vi"("Aktionen"=Aktionen_Polynom_Daten_speichern."lesen") -> ("Aktiv"=w597:bool[], "Namen"=w587:string[])  [unwired: 5 in, 4 out]
      n407 = call "FGV Gasliste.vi"("Aktionen"=FGV_FT-IR_Gasliste_Aktionen."laden") -> ("Aktuelle Gasliste gesamt"=w589:T48[])  [unwired: 8 in, 2 out]
      n408 = local write "Status"(w570) -> ()
      n409 = call "FGV Daten Abholung uebergeben.vi"("Zustand"=w570, "Beendet"=FALSE, "Aktion"=Aktion_FGV_Daten_Abholung_uebergebenctl."schreiben") -> ()  [unwired: 8 in, 5 out]
      n410 = Build Array(w589, w587) -> (w588:T48[][])
      n411 = Build Array (concatenate)("----", w589) -> ()  [unwired: 1 out]
      n412 = local write "PolynomAktiv"(w597) -> ()
      n413 = property on="Stufen Tabelle" class="Tbl (strikt)"("DisabledEnum"=w621) -> (error out=w601:errorcluster)  [unwired: 2 in, 1 out]
      n414 = property on="Abfragen" class="Bool."("DisabledEnum"=w621) -> (error out=w600:errorcluster)  [unwired: 2 in, 1 out]
      n415 = Unbundle By Name(w622) -> ("Gasteiler"=w590:T12, "Gasteiler Type"=w541:T15)
      n416 = local write "Serielle Parameter"(w585) -> ()
      n417 = Unbundle By Name(w618) -> ("IP-Adresse"=w617:string, "Aktive"=w606:bool, "Port"=w605:u16)
      n418 = Transpose 2D Array(2D array=w588) -> (transposed array=→"PolynomTabelleAnzeige":T48[][])
      n419 = local write "Port"(w605) -> ()
      n420 = local write "TCP Verbindung aktiv"(w606) -> ()
      n421 = Merge Errors(w601, w600) -> (w599:errorcluster)
      n422 = for {
        N: 4 -> [_]
        shift-right: [w634] -> _
        shift-left: w617 -> [w637]
        tunnel: [w633] -> w616 mode=indexing
        n423 = Search/Split String(string=w637, search string/char (-)="." ("Nach String/Zeichen suchen (-)")) -> (substring before match=w633:string, match + rest of string=w636:string)  [unwired: 1 in, 1 out]
        n424 = String Subset(string=w636, offset (0)=1 ("Offset (0)")) -> (substring=w634:string)  [unwired: 1 in]
      }
      n425 = property on="automatisch" class="Bool. (strikt)"("Visible"=w519) -> (error out=w528:errorcluster)  [unwired: 2 in, 1 out]
      n426 = local write "Pfad Auto Lin"(w518) -> ()
      n427 = local write "Pfad LIN"(w518) -> ()
      n428 = local write "EPA Pfad"(w518) -> ()
      n429 = property on="PDF single pages Span" class="Bool. (strikt)"("Visible"=w519) -> (error out=w530:errorcluster)  [unwired: 2 in, 1 out]
      n430 = property on="PDF Deckblatt" class="Bool. (strikt)"("Visible"=FALSE ("Sichtbar")) -> (error out=w525:errorcluster)  [unwired: 2 in, 1 out]
      n431 = property on="Pfad Auto Lin" class="Pfad (strikt)"("Visible"=w519) -> ()  [unwired: 2 in, 2 out]
      n432 = call <vilib>:"Clear Errors.vi"("error in (no error)"=w599) -> ()  [unwired: 5 in, 2 out]
      n433 = Merge Errors(w528, w530, w525) -> (w529:errorcluster)
      n434 = control-ref of="automatisch"() -> (w549:refnum<vi>)
      n435 = call "Lin Daten aufarbeiten.vi"("Aktionen"=Aktion_Lin_Daten_aufarbeiten."lesen") -> ("Lin-Polynom"=w592:T119)  [unwired: 16 in, 10 out]
      n436 = call <vilib>:"Clear Errors.vi"("error in (no error)"=w529) -> ()  [unwired: 5 in, 2 out]
      n437 = control-ref of="Gasteiler Span Eingänge"() -> (w548:refnum<vi>)
      n438 = Index Array(array=w616) -> (element #1=w615:string, element #2=w614:string, element #3=w613:string, element #4=w612:string)  [unwired: 4 in]
      n439 = Bundle By Name(cluster=w592, "Kalibrator (Gasteiler)"=w590) -> (w594:T119)
      n440 = call "Span Register setzen.vi"("init"=w531, "error in (no error)"=w544, "GD Span Eingänge"=w548, "automatisch Boolesch (Eingang)"=w549) -> ("GD Span Eingänge out"=w547:refnum<vi>, "automatisch Boolesch (Ausgang)"=w546:refnum<vi>, "automatisch out"=w545:T20, "auto Deaktiviert"=w533:T66, "GD Span Eingänge"=w543:u16)  [unwired: 1 in, 2 out]
      n441 = Decimal String To Number(string=w615, default (0L)=w611) -> (number=w610:u8)  [unwired: 1 in, 1 out]
      n442 = Decimal String To Number(string=w614, default (0L)=w611) -> (number=w608:u8)  [unwired: 1 in, 1 out]
      n443 = Decimal String To Number(string=w613, default (0L)=w611) -> (number=w607:u8)  [unwired: 1 in, 1 out]
      n444 = Decimal String To Number(string=w612, default (0L)=w611) -> (number=w609:u8)  [unwired: 1 in, 1 out]
      n445 = local write "IP 1"(w610) -> ()
      n446 = local write "IP 2"(w608) -> ()
      n447 = local write "IP 3"(w607) -> ()
      n448 = local write "IP 4"(w609) -> ()
      n449 = local read "automatisch"() -> (w552:T1)
      n450 = call "Lin Daten aufarbeiten.vi"("Lin-Polynom"=w594, "Aktionen"=Aktion_Lin_Daten_aufarbeiten."Protkolldaten") -> ()  [unwired: 15 in, 11 out]
      n451 = Equal?(x=w579, y=w541) -> (x = y?=w534:bool)
      n452 = Not Equal?(x=w541, y=w540) -> (x != y?=w538:bool)
      n453 = Not Equal?(x=w541, y=w539) -> (x != y?=w537:bool)
      n454 = local write "Gasnummer HovaCal Interface"(w568) -> ()
      n455 = And(x=w538, y=w537) -> (x .and. y?=w535:bool)
      n456 = property on="Gasnummer Generieren" class="DigWert (strikt)"("Val(Sgnl)"=w568) -> (error out=w596:errorcluster)  [unwired: 2 in, 1 out]
      n457 = local write "Gasnummer Generieren"(w568) -> ()
      n458 = local write "Gasnummer HovaCal"(w568) -> ()
      n459 = Not(x=w534) -> (.not. x?=w574:bool)
      n460 = local write "Gasnummer EPA"(w568) -> ()
      n461 = local write "Gasnummer LIN"(w568) -> ()
      n462 = call "FGV Gasteilerkorrektur.vi"("Aktion"=Aktion_FGV_Gasteiler_Korrektur."laden") -> ()  [unwired: 9 in, 6 out]
